vi "UNBILITZ-ShutterDriver-Close.vi"(0 "VISA resource name":refnum<visa-resource-name>, 11 "error in (no error)":errorcluster) -> (15 "error out":errorcluster)   [LabVIEW 2012]
doc: "Closes the serial connection to the Uniblitz shutter driver device."
panel:
  # "Inputs"
  # "Outputs"
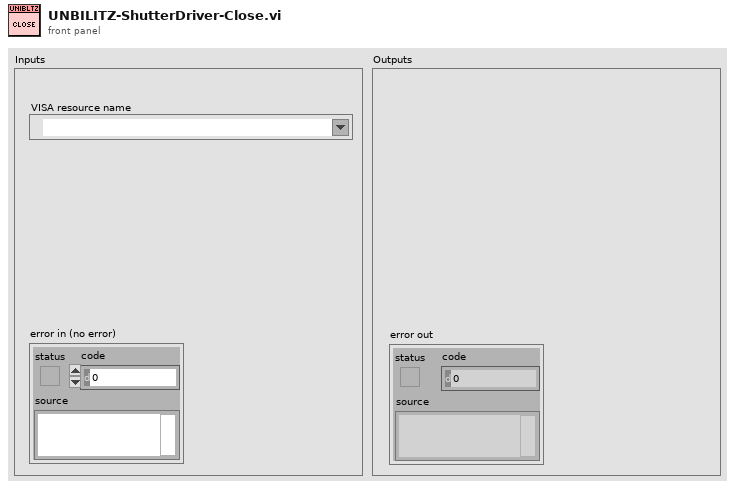
[diagram p1: front panel]
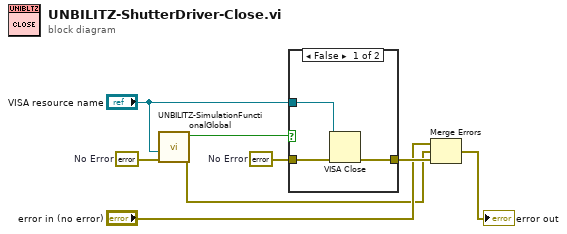
[diagram p0: block diagram]
diagram:
  w1 = errorcluster {"status"=FALSE, "code"=0, "source"=""}  # No Error
  w4 = errorcluster {"status"=FALSE, "code"=0, "source"=""}  # No Error
  n1 = call "UNBILITZ-SimulationFunctionalGlobal.vi"("error in (no error)"=w4, "VISA Resource Name"="VISA resource name") -> ("error out"=w2:errorcluster, "Simulation Mode"=w6:bool)  [unwired: 8 in]
  n2 = case shown="False" w6 {
    tunnel: w1 -> [w9 w12]
    tunnel: [w11 w12] -> w8
    tunnel: "VISA resource name" -> [w10 _]
    frame False {
      n3 = VISA Close(VISA resource name=w10, error in (no error)=w9) -> (error out=w11:errorcluster)
    }
    frame True {
    }
  }
  n4 = Merge Errors("error in (no error)", w2, w8) -> (→"error out":errorcluster)
